vi "ANALIZA.vi"(11 "Array":dbl[](array[numeric])) -> (1 "Odchylenie standardowe":dbl, 2 "Wariancja":dbl, 3 "Œrednia arytmetyczna":dbl)   [LabVIEW 2025]
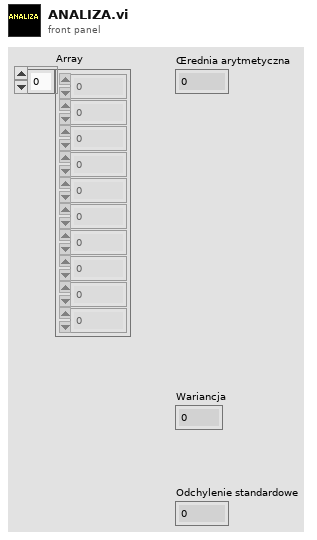
[diagram p1: front panel]
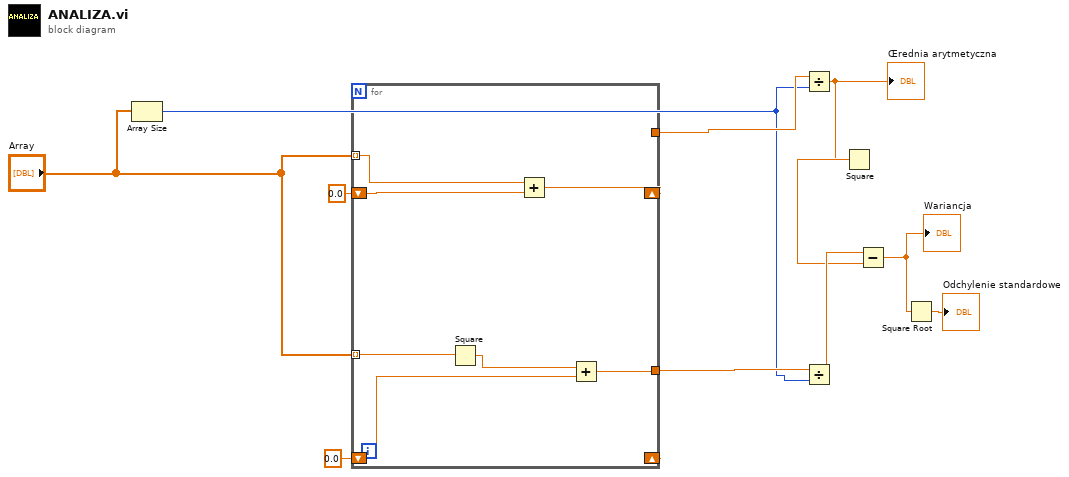
[diagram p0: block diagram]
diagram:
  n1 = Array Size(array="Array") -> (size(s)=w1:i32)
  n2 = for {
    tunnel: "Array" -> [w17] mode=indexing
    shift-right: [w16] -> _
    shift-left: 0.0 -> [w18]
    tunnel: [w16] -> w5
    tunnel: "Array" -> [w15] mode=indexing
    shift-right: [w12] -> _
    shift-left: 0.0 -> [w13]
    tunnel: [w12] -> w2
    n3 = Square(x=w15) -> (x^2=w14:dbl)
    n4 = Add(x=w17, y=w18) -> (x+y=w16:dbl)
    n5 = Add(x=w14, y=w13) -> (x+y=w12:dbl)
  }
  n6 = Divide(x=w5, y=w1) -> (x/y=w7:dbl)
  "Œrednia arytmetyczna" <- w7
  n7 = Divide(x=w2, y=w1) -> (x/y=w9:dbl)
  n8 = Square(x=w7) -> (x^2=w8:dbl)
  n9 = Subtract(x=w9, y=w8) -> (x-y=w10:dbl)
  "Wariancja" <- w10
  n10 = Square Root(x=w10) -> (sqrt(x)=→"Odchylenie standardowe":dbl)
